vi "6509_read.vi"(8 "error in":errorcluster, 11 "task in":refnum<k21>) -> (0 "error out":errorcluster, 2 "edge":cluster{"itrp":bool[], "time":dbl}, 3 "task out":refnum<k21>)   [LabVIEW 2018, in "6509.lvlib"]
uses:
  Libraries/6509/6509.lvlib
  <vilib>/DAQmx/read.llb/DAQmx Read (Digital 1D Bool NChan 1Samp 1Line).vi
  <vilib>/DAQmx/miscellaneous.llb/DAQmx Fill In Error Info.vi
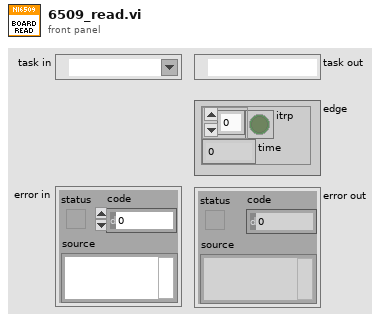
[diagram p1: front panel]
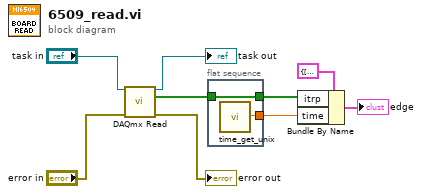
[diagram p0: block diagram]
diagram:
  n1 = call-poly <vilib>:"DAQmx Read.vi"("task/channels in"="task in", "error in"="error in") -> ("task out"=→"task out":refnum<k21>, "data"=w5:bool[], "error out"=→"error out":errorcluster)  [unwired: 11 in]
  n2 = flat-sequence {
    tunnel: [w10] -> w2
    tunnel: w5 -> [w11]
    tunnel: [w11] -> w4
    frame #0 {
      n3 = call "time_get_unix.vi"() -> ("unix_timestamp"=w10:dbl)
    }
  }
  n4 = Bundle By Name(cluster=cluster{"itrp":bool[], "time":dbl} {"itrp"=[], "time"=0.0} ("edge"), "itrp"=w4, "time"=w2) -> (→"edge":cluster{"itrp":bool[], "time":dbl})
